vi "WPI_CANJaguar_ConfigLimits.vi"(0 "CAN Jaguar Ref":T2={"DeviceStatus"={"status"=FALSE, "code"=0, "source"=""}, "Type"=enum."PWM", "PWM"={"PWM Channel"=enum."PWM 1", "DeadBand"={"Name"="", "maxPositivePwm"=0, "minPositivePwm"=0, "centerPwm"=0, "maxNegativePwm"=0, "minNegativePwm"=0, "angularRange"=0}}, "CAN"={"Device Number"=0, "SetOutput VI Ref"=variant(enum8{"Percent VBus", "Current", "Speed", "Position", "Voltage"} enum."Percent VBus"), "GetOutput VI Ref"=variant(refnum<k1> refnum), "Enable VI Ref"=variant(dbl 12.0), "Disable VI Ref"=variant(enum8{"Percent VBus", "Speed", "Position", "Slave", "Unchanged / Invalid", "Voltage Compensation", "Current", "Motion Profile"} enum."Percent VBus"), "Data"=variant}, "Invert"=FALSE}, 5 "Limit Mode":T1, 7 "Forward Limit Position":dbl, 9 "Reverse Limit Position":dbl, 11 "error in (no error)":errorcluster) -> (4 "CAN Jaguar Ref":T2={"DeviceStatus"={"status"=FALSE, "code"=0, "source"=""}, "Type"=enum."PWM", "PWM"={"PWM Channel"=enum."PWM 1", "DeadBand"={"Name"="", "maxPositivePwm"=0, "minPositivePwm"=0, "centerPwm"=0, "maxNegativePwm"=0, "minNegativePwm"=0, "angularRange"=0}}, "CAN"={"Device Number"=0, "SetOutput VI Ref"=variant(enum8{"Percent VBus", "Current", "Speed", "Position", "Voltage"} enum."Percent VBus"), "GetOutput VI Ref"=variant(refnum<k1> refnum), "Enable VI Ref"=variant(dbl 12.0), "Disable VI Ref"=variant(enum8{"Percent VBus", "Speed", "Position", "Slave", "Unchanged / Invalid", "Voltage Compensation", "Current", "Motion Profile"} enum."Percent VBus"), "Data"=variant}, "Invert"=FALSE}, 15 "error out":errorcluster)   [LabVIEW 2016]
doc: "Configure how the limits in Jaguar function. If in <B>Position</B> control mode, additional soft limits can be enabled. The wired limit switch inputs are always active and cannot be disabled."
uses:
  <vilib>/Rock Robotics/WPI/MotorControl/WPI_MotorControlDeviceRef.ctl
  <vilib>/Rock Robotics/WPI/MotorControl/WPI_MotorControlType.ctl
  <vilib>/Rock Robotics/SystemInterfaces/DIO/FPGA_DIOPWMChannel.ctl
  <vilib>/Rock Robotics/WPI/PWM/WPI_PWMDeadband.ctl
  <vilib>/Rock Robotics/WPI/ThirdParty/CanMotor/CAN Jaguar/SubVIs/WPI_CANJaguar_LimitMode.ctl
  <vilib>/Rock Robotics/WPI/ThirdParty/CanMotor/CAN Jaguar/SubVIs/WPI_CAN_MotorMessageIDs.ctl
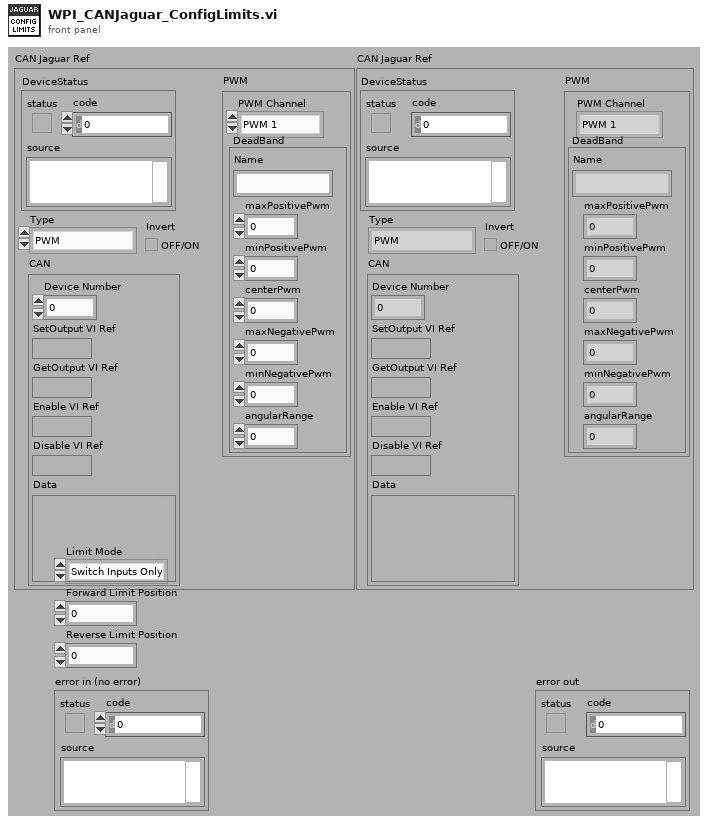
[diagram p1: front panel]
types:
  T1 = typedef "WPI_CANJaguar_LimitMode.ctl" = enum16{"Switch Inputs Only", "Soft Position Limits"}
  T2 = typedef "WPI_MotorControlDeviceRef.ctl" = cluster{"DeviceStatus":errorcluster, "Type":T3, "PWM":cluster{"PWM Channel":T4, "DeadBand":T5}, "CAN":cluster{"Device Number":u8, "SetOutput VI Ref":variant, "GetOutput VI Ref":variant, "Enable VI Ref":variant, "Disable VI Ref":variant, "Data":variant}, "Invert":bool}
  T3 = typedef "WPI_MotorControlType.ctl" = enum16{"PWM", "CAN"}
  T4 = typedef "FPGA_DIOPWMChannel.ctl" = enum8{"PWM 0", "PWM 1", "PWM 2", "PWM 3", "PWM 4", "PWM 5", "PWM 6", "PWM 7", "PWM 8", "PWM 9", "PWM MXP 0", "PWM MXP 1", "PWM MXP 2", "PWM MXP 3", "PWM MXP 4", "PWM MXP 5", "PWM MXP 6", "PWM MXP 7", "PWM MXP 8", "PWM MXP 9", "Invalid"}
  T5 = typedef "WPI_PWMDeadband.ctl" = cluster{"Name":string, "maxPositivePwm":i32, "minPositivePwm":i32, "centerPwm":i32, "maxNegativePwm":i32, "minNegativePwm":i32, "angularRange":u16}
  T6 = enum16{"big-endian, network order", "native, host order", "little-endian"}
  T7 = typedef "WPI_CAN_MotorMessageIDs.ctl" = u32
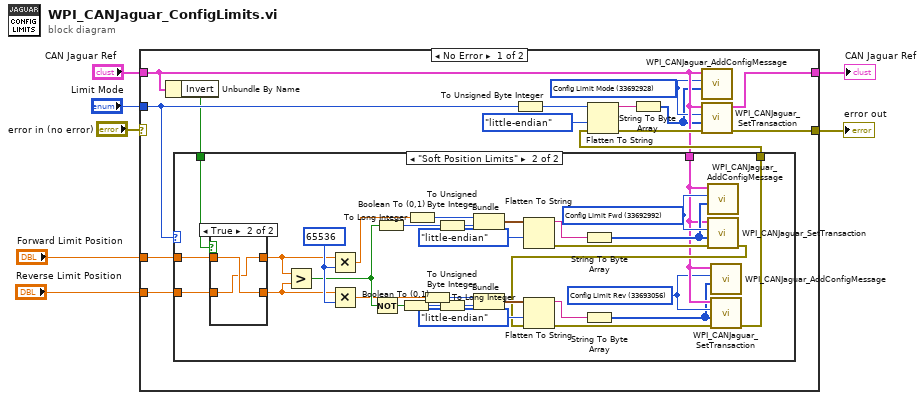
[diagram p0: block diagram]
diagram:
  n1 = case shown="No Error" "error in (no error)" {
    selector: "error in (no error)" -> [_ w58]
    tunnel: [w12 w58] -> w7
    tunnel: [w13 w57] -> w5
    tunnel: "CAN Jaguar Ref" -> [w10 w57]
    tunnel: "Limit Mode" -> [w18 _]
    tunnel: "Forward Limit Position" -> [w17 _]
    tunnel: "Reverse Limit Position" -> [w16 _]
    frame No Error {
      w9 = T7 33692928 items=["Volt Enable"=33685504, "Volt Disable"=33685568, "Volt Set"=33685632, "Volt Set Ramp"=33685696, "Speed Enable"=33686528, "Speed Disable"=33686592, "Speed Set"=33686656, "Speed P"=33686720, "Speed I"=33686784, "Speed D"=33686848, "Speed Ref"=33686912, "Volt Comp Enable"=33687552, "Volt Comp Disable"=33687616, "Volt Comp Set"=33687680, "Volt Comp In Ramp"=33687744, "Volt Comp Comp Ramp"=33687808, "Position Enable"=33688576, "Position Disable"=33688640, "Position Set"=33688704, "Position P"=33688768, "Position I"=33688832, "Position D"=33688896, "Position Ref"=33688960, "Current Enable"=33689600, "Current Disable"=33689664, "Current Set"=33689728, "Current P"=33689792, "Current I"=33689856, "Current D"=33689920, "Status Percent VBus"=33690624, "Status VBus"=33690688, "Status Current"=33690752, "Status Temp"=33690816, "Status Position"=33690880, "Status Speed"=33690944, "Status Limit"=33691008, "Status Fault"=33691072, "Status Power"=33691136, "Status Control Mode"=33691200, "Status VOut"=33691264, "Config Num Brushes"=33692672, "Config Encoder Lines"=33692736, "Config Pot Turns"=33692800, "Config Brake Coast"=33692864, "Config Limit Mode"=33692928, "Config Limit Fwd"=33692992, "Config Limit Rev"=33693056, "Config Max VOut"=33693120, "Config Fault Time"=33693184, "Motor Ack"=33693696] ("CAN Motor Message IDs")
      n2 = Unbundle By Name(w10) -> ("Invert"=w11:bool)
      n3 = case shown="\"Soft Position Limits\"" w18 {
        tunnel: w17 -> [_ w30]
        tunnel: w16 -> [_ w28]
        tunnel: [_ w32] -> w15
        tunnel: w10 -> [_ w24]
        tunnel: w11 -> [_ w31]
        frame Default {
        }
        frame "Soft Position Limits" {
          w23 = T7 33693056 items=["Volt Enable"=33685504, "Volt Disable"=33685568, "Volt Set"=33685632, "Volt Set Ramp"=33685696, "Speed Enable"=33686528, "Speed Disable"=33686592, "Speed Set"=33686656, "Speed P"=33686720, "Speed I"=33686784, "Speed D"=33686848, "Speed Ref"=33686912, "Volt Comp Enable"=33687552, "Volt Comp Disable"=33687616, "Volt Comp Set"=33687680, "Volt Comp In Ramp"=33687744, "Volt Comp Comp Ramp"=33687808, "Position Enable"=33688576, "Position Disable"=33688640, "Position Set"=33688704, "Position P"=33688768, "Position I"=33688832, "Position D"=33688896, "Position Ref"=33688960, "Current Enable"=33689600, "Current Disable"=33689664, "Current Set"=33689728, "Current P"=33689792, "Current I"=33689856, "Current D"=33689920, "Status Percent VBus"=33690624, "Status VBus"=33690688, "Status Current"=33690752, "Status Temp"=33690816, "Status Position"=33690880, "Status Speed"=33690944, "Status Limit"=33691008, "Status Fault"=33691072, "Status Power"=33691136, "Status Control Mode"=33691200, "Status VOut"=33691264, "Config Num Brushes"=33692672, "Config Encoder Lines"=33692736, "Config Pot Turns"=33692800, "Config Brake Coast"=33692864, "Config Limit Mode"=33692928, "Config Limit Fwd"=33692992, "Config Limit Rev"=33693056, "Config Max VOut"=33693120, "Config Fault Time"=33693184, "Motor Ack"=33693696] ("CAN Motor Message IDs")
          w49 = 65536
          w26 = T7 33692992 items=["Volt Enable"=33685504, "Volt Disable"=33685568, "Volt Set"=33685632, "Volt Set Ramp"=33685696, "Speed Enable"=33686528, "Speed Disable"=33686592, "Speed Set"=33686656, "Speed P"=33686720, "Speed I"=33686784, "Speed D"=33686848, "Speed Ref"=33686912, "Volt Comp Enable"=33687552, "Volt Comp Disable"=33687616, "Volt Comp Set"=33687680, "Volt Comp In Ramp"=33687744, "Volt Comp Comp Ramp"=33687808, "Position Enable"=33688576, "Position Disable"=33688640, "Position Set"=33688704, "Position P"=33688768, "Position I"=33688832, "Position D"=33688896, "Position Ref"=33688960, "Current Enable"=33689600, "Current Disable"=33689664, "Current Set"=33689728, "Current P"=33689792, "Current I"=33689856, "Current D"=33689920, "Status Percent VBus"=33690624, "Status VBus"=33690688, "Status Current"=33690752, "Status Temp"=33690816, "Status Position"=33690880, "Status Speed"=33690944, "Status Limit"=33691008, "Status Fault"=33691072, "Status Power"=33691136, "Status Control Mode"=33691200, "Status VOut"=33691264, "Config Num Brushes"=33692672, "Config Encoder Lines"=33692736, "Config Pot Turns"=33692800, "Config Brake Coast"=33692864, "Config Limit Mode"=33692928, "Config Limit Fwd"=33692992, "Config Limit Rev"=33693056, "Config Max VOut"=33693120, "Config Fault Time"=33693184, "Motor Ack"=33693696] ("CAN Motor Message IDs")
          n4 = case shown="True" w31 {
            tunnel: [w54 w55] -> w29
            tunnel: w30 -> [w54 w56]
            tunnel: [w53 w56] -> w27
            tunnel: w28 -> [w53 w55]
            frame False {
            }
            frame True {
            }
          }
          n5 = Greater?(x=w29, y=w27) -> (0:w44:bool)
          n6 = Multiply(x=w29, y=w49) -> (x*y=w47:dbl)
          n7 = Multiply(x=w27, y=w49) -> (x*y=w37:dbl)
          n8 = Not(x=w44) -> (.not. x?=w36:bool)
          n9 = Boolean To (0,1)(Boolean=w44) -> (0, 1=w46:i16)
          n10 = Boolean To (0,1)(Boolean=w36) -> (0, 1=w42:i16)
          n11 = To Long Integer(number=w47) -> (32bit integer=w48:i32)
          n12 = To Long Integer(number=w37) -> (32bit integer=w41:i32)
          n13 = To Unsigned Byte Integer(number=w46) -> (unsigned 8bit integer=w45:u8)
          n14 = To Unsigned Byte Integer(number=w42) -> (unsigned 8bit integer=w43:u8)
          n15 = Bundle(w48, w45) -> (w50:cluster{i32, u8})  [unwired: 1 out]
          n16 = Bundle(w41, w43) -> (w40:cluster{i32, u8})  [unwired: 1 out]
          n17 = Flatten To String(anything=w50, byte order (0:big-endian, network order)=T6."little-endian") -> (data string=w52:string, error out=w35:errorcluster)  [unwired: 1 in, 2 out]
          n18 = String To Byte Array(string=w52) -> (unsigned byte array=w25:u8[])
          n19 = call <vilib>:"WPI_CANJaguar_AddConfigMessage.vi"("Data"=w25, "Message ID"=w26, "CAN Jaguar Ref"=w24) -> ()  [unwired: 9 in]
          n20 = call <vilib>:"WPI_CANJaguar_SetTransaction.vi"("error in"=w35, "Data"=w25, "Message ID"=w26, "CAN Jaguar Ref"=w24) -> ("error out"=w34:errorcluster)  [unwired: 7 out]
          n21 = Flatten To String(anything=w40, byte order (0:big-endian, network order)=T6."little-endian", error in (no error)=w34) -> (data string=w38:string, error out=w33:errorcluster)  [unwired: 2 out]
          n22 = String To Byte Array(string=w38) -> (unsigned byte array=w22:u8[])
          n23 = call <vilib>:"WPI_CANJaguar_AddConfigMessage.vi"("Data"=w22, "Message ID"=w23, "CAN Jaguar Ref"=w24) -> ()  [unwired: 9 in]
          n24 = call <vilib>:"WPI_CANJaguar_SetTransaction.vi"("error in"=w33, "Data"=w22, "Message ID"=w23, "CAN Jaguar Ref"=w24) -> ("error out"=w32:errorcluster)  [unwired: 7 out]
        }
      }
      n25 = To Unsigned Byte Integer(number=w18) -> (unsigned 8bit integer=w19:u8)
      n26 = Flatten To String(anything=w19, byte order (0:big-endian, network order)=T6."little-endian", error in (no error)=w15) -> (data string=w20:string, error out=w14:errorcluster)  [unwired: 2 out]
      n27 = String To Byte Array(string=w20) -> (unsigned byte array=w8:u8[])
      n28 = call <vilib>:"WPI_CANJaguar_AddConfigMessage.vi"("Data"=w8, "Message ID"=w9, "CAN Jaguar Ref"=w10) -> ()  [unwired: 9 in]
      n29 = call <vilib>:"WPI_CANJaguar_SetTransaction.vi"("error in"=w14, "Data"=w8, "Message ID"=w9, "CAN Jaguar Ref"=w10) -> ("error out"=w12:errorcluster, "CAN Jaguar Ref Out"=w13:T2)  [unwired: 6 out]
    }
    frame Error {
    }
  }
  "CAN Jaguar Ref" <- w5
  "error out" <- w7
